vi "FilterByMatchingString.vi"(6 "AND Condition?":bool, 8 "error in (no error)":errorcluster, 9 "Target filter":refnum<class "CItemMatch.lvclass">, 10 "Source filter":refnum<class "CItemMatch.lvclass">, 11 "CDependencyList in":refnum<class "CDependencyList.lvclass">) -> (0 "error out":errorcluster, 3 "CDependencyList out":refnum<class "CDependencyList.lvclass">)   [LabVIEW 2020, in "DependencyInspection.lvlib" / "CDependencyList.lvclass"]
uses:
  CDependencyList.lvclass
  LabVIEWObjectInterfaces/ILabVIEWItem/ILabVIEWItem.lvclass
  LabVIEWObjectFactory/LabVIEWObjectFactory.lvlib
  CItemMatch/CItemMatch.lvclass
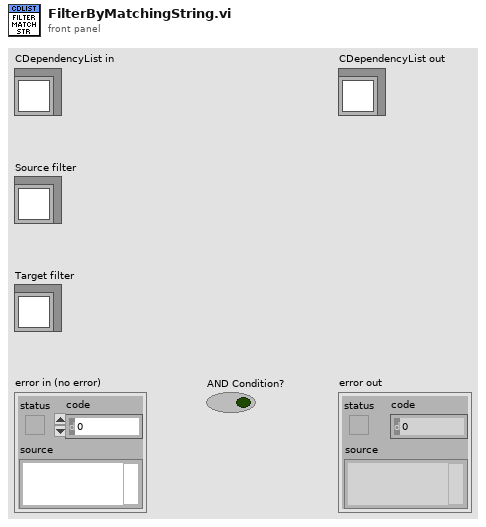
[diagram p1: front panel]
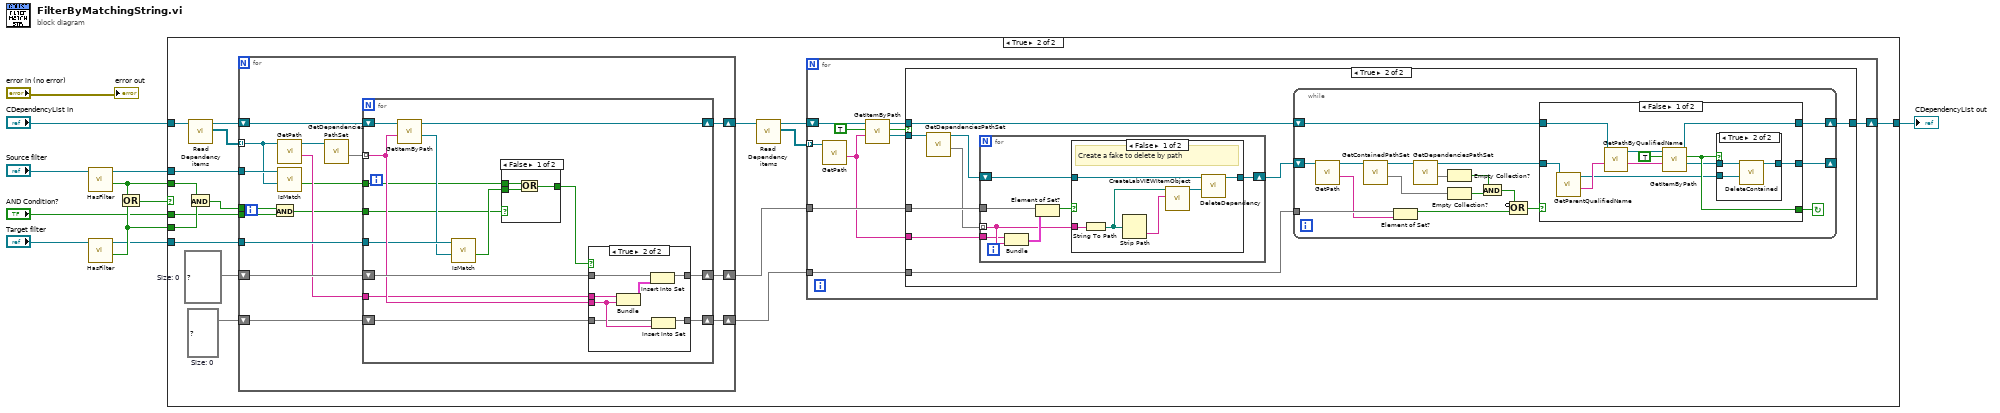
[diagram p0: block diagram]
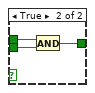
[diagram p3: hidden frame]
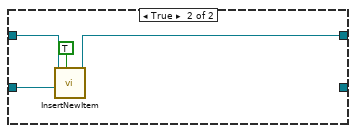
[diagram p8: hidden frame]
diagram:
  n1 = call-dynamic "HasFilter.vi"("CItemMatch in"="Source filter") -> ("Has filter?"=w7:bool, "CItemMatch out"=w5:refnum<class "CItemMatch.lvclass">)  [unwired: 8 in, 1 out]
  n2 = call-dynamic "HasFilter.vi"("CItemMatch in"="Target filter") -> ("Has filter?"=w4:bool, "CItemMatch out"=w2:refnum<class "CItemMatch.lvclass">)  [unwired: 8 in, 1 out]
  n3 = Or(x=w7, y=w4) -> (x .or. y?=w8:bool)
  n4 = case shown="True" w8 {
    tunnel: "CDependencyList in" -> [w12 w29]
    tunnel: w2 -> [_ w25]
    tunnel: w5 -> [_ w24]
    tunnel: [w12 w19] -> w9
    tunnel: w7 -> [_ w18]
    tunnel: w4 -> [_ w17]
    tunnel: "AND Condition?" -> [_ w13]
    frame False {
    }
    frame True {
      w16 = set{string} {}  # Size: 0
      w23 = set{cluster{"Source":string, "Target":string}} {}  # Size: 0
      n5 = call-dynamic "Read Dependency items.vi"("CDependencyList in"=w29) -> ("Dependency items"=w28:refnum<class "ILabVIEWItem.lvclass">[], "CDependencyList out"=w27:refnum<class "CDependencyList.lvclass">)  [unwired: 9 in]
      n6 = And(x=w18, y=w17) -> (x .and. y?=w14:bool)
      n7 = for {
        tunnel: w28 -> [w37] mode=indexing
        shift-right: [w43] -> w26
        shift-left: w27 -> [w45]
        tunnel: w25 -> [w44]
        tunnel: w24 -> [w38]
        shift-right: [w42] -> w20
        shift-left: w23 -> [w41]
        shift-right: [w40] -> w15
        shift-left: w16 -> [w39]
        tunnel: w14 -> [w30]
        tunnel: w13 -> [w32]
        n8 = And(x=w30, y=w32) -> (x .and. y?=w31:bool)
        n9 = call-dynamic "GetPath.vi"("ILabVIEWItem in"=w37) -> ("Path"=w34:string, "ILabVIEWItem out"=w35:refnum<class "ILabVIEWItem.lvclass">)  [unwired: 8 in, 1 out]
        n10 = call-dynamic "IsMatch.vi"("Item to match"=w37, "CItemMatch in"=w38) -> ("Is match?"=w33:bool)  [unwired: 7 in, 2 out]
        n11 = call-dynamic "GetDependenciesPathSet.vi"("ILabVIEWItem in"=w35) -> ("Dependencies"=w36:set{string})  [unwired: 8 in, 2 out]
        n12 = for {
          tunnel: w36 -> [w55] mode=indexing
          shift-right: [w58] -> w43
          shift-left: w45 -> [w59]
          tunnel: w44 -> [w51]
          shift-right: [w56] -> w42
          shift-left: w41 -> [w57]
          tunnel: w34 -> [w54]
          shift-right: [w53] -> w40
          shift-left: w39 -> [w52]
          tunnel: w33 -> [w48]
          tunnel: w31 -> [w47]
          n13 = call-dynamic "GetItemByPath.vi"("Path"=w55, "CDependencyList in"=w59) -> ("ILabVIEWItem"=w50:refnum<class "ILabVIEWItem.lvclass">, "CDependencyList out"=w58:refnum<class "CDependencyList.lvclass">)  [unwired: 6 in, 2 out]
          n14 = call-dynamic "IsMatch.vi"("Item to match"=w50, "CItemMatch in"=w51) -> ("Is match?"=w49:bool)  [unwired: 7 in, 2 out]
          n15 = case shown="False" w47 {
            tunnel: w49 -> [w62 w64]
            tunnel: w48 -> [w61 w65]
            tunnel: [w60 w63] -> w46
            frame False {
              n16 = Or(x=w61, y=w62) -> (x .or. y?=w60:bool)
            }
            frame True {
              n17 = And(x=w65, y=w64) -> (x .and. y?=w63:bool)
            }
          }
          n18 = case shown="True" w46 {
            tunnel: w57 -> [w67 w73]
            tunnel: [w67 w74] -> w56
            tunnel: w55 -> [_ w70]
            tunnel: w54 -> [_ w72]
            tunnel: [w66 w69] -> w53
            tunnel: w52 -> [w66 w68]
            frame False {
            }
            frame True {
              n19 = Bundle("Path"=w72, "Path"=w70) -> (w71:cluster{"Path":string, "Path":string})  [unwired: 1 in]
              n20 = Insert Into Set(10:w71, 11:w73) -> (3:w74:set{cluster{"Source":string, "Target":string}})  [unwired: 1 out]
              n21 = Insert Into Set(10:w70, 11:w68) -> (3:w69:set{string})  [unwired: 1 out]
            }
          }
        }
      }
      n22 = call-dynamic "Read Dependency items.vi"("CDependencyList in"=w26) -> ("Dependency items"=w21:refnum<class "ILabVIEWItem.lvclass">[], "CDependencyList out"=w22:refnum<class "CDependencyList.lvclass">)  [unwired: 9 in]
      n23 = for {
        shift-right: [w79] -> w19
        shift-left: w22 -> [w83]
        tunnel: w21 -> [w82] mode=indexing
        tunnel: w20 -> [w78]
        tunnel: w15 -> [w75]
        n24 = call-dynamic "GetPath.vi"("ILabVIEWItem in"=w82) -> ("Path"=w76:string)  [unwired: 8 in, 2 out]
        n25 = call-dynamic "GetItemByPath.vi"("Path"=w76, "Remove?"=TRUE, "CDependencyList in"=w83) -> ("ILabVIEWItem"=w80:refnum<class "ILabVIEWItem.lvclass">, "key found?"=w77:bool, "CDependencyList out"=w81:refnum<class "CDependencyList.lvclass">)  [unwired: 5 in, 1 out]
        n26 = case shown="True" w77 {
          tunnel: w81 -> [w85 w90]
          tunnel: w80 -> [_ w93]
          tunnel: [w85 w94] -> w79
          tunnel: w78 -> [_ w91]
          tunnel: w76 -> [_ w87]
          tunnel: w75 -> [_ w86]
          frame False {
          }
          frame True {
            n27 = call-dynamic "GetDependenciesPathSet.vi"("ILabVIEWItem in"=w93) -> ("Dependencies"=w89:set{string}, "ILabVIEWItem out"=w88:refnum<class "ILabVIEWItem.lvclass">)  [unwired: 8 in, 1 out]
            n28 = for {
              tunnel: w89 -> [w96] mode=indexing
              tunnel: w91 -> [w101]
              shift-right: [w98] -> w92
              shift-left: w88 -> [w99]
              tunnel: w87 -> [w95]
              n29 = Bundle("Path"=w95, "Path"=w96) -> (w97:cluster{"Path":string, "Path":string})  [unwired: 1 in]
              n30 = Element of Set?(10:w97, 11:w101) -> (3:w100:bool)
              n31 = case shown="False" w100 {
                tunnel: w99 -> [w107 w108]
                tunnel: [w106 w108] -> w98
                tunnel: w96 -> [w104 _]
                frame False {
                  # "Create a fake to delete by path"
                  n32 = String To Path(string=w104) -> (path=w102:path)
                  n33 = Strip Path(path=w102) -> (name=w103:string)  [unwired: 1 out]
                  n34 = call "CreateLabVIEWItemObject.vi"("delimited name"=w103, "SubVI path"=w102) -> ("ILabVIEWItem"=w105:refnum<class "ILabVIEWItem.lvclass">)  [unwired: 8 in, 1 out]
                  n35 = call-dynamic "DeleteDependency.vi"("Item to depend on"=w105, "ILabVIEWItem in"=w107) -> ("ILabVIEWItem out"=w106:refnum<class "ILabVIEWItem.lvclass">)  [unwired: 8 in, 1 out]
                }
                frame True {
                }
              }
            }
            n36 = while {
              shift-right: [w120] -> w94
              shift-left: w90 -> [w123]
              shift-right: [w119] -> _
              shift-left: w92 -> [w117]
              tunnel: w86 -> [w115]
              stop <- w118 continue-if-true
              n37 = call-dynamic "GetPath.vi"("ILabVIEWItem in"=w117) -> ("Path"=w110:string, "ILabVIEWItem out"=w116:refnum<class "ILabVIEWItem.lvclass">)  [unwired: 8 in, 1 out]
              n38 = call-dynamic "GetContainedPathSet.vi"("ILabVIEWItem in"=w116) -> ("Contained"=w121:set{string}, "ILabVIEWItem out"=w122:refnum<class "ILabVIEWItem.lvclass">)  [unwired: 8 in, 1 out]
              n39 = Element of Set?(10:w110, 11:w115) -> (3:w112:bool)
              n40 = call-dynamic "GetDependenciesPathSet.vi"("ILabVIEWItem in"=w122) -> ("Dependencies"=w125:set{string}, "ILabVIEWItem out"=w124:refnum<class "ILabVIEWItem.lvclass">)  [unwired: 8 in, 1 out]
              n41 = Empty Collection?(1:w125) -> (0:w113:bool)
              n42 = Empty Collection?(1:w121) -> (0:w114:bool)
              n43 = And(x=w113, y=w114) -> (x .and. y?=w111:bool)
              n44 = Compound Arithmetic op=OR(invert w111, w112) -> (w109:bool)
              n45 = case shown="False" w109 {
                tunnel: w124 -> [w128 w142]
                tunnel: w123 -> [w127 w143]
                tunnel: [w126 w141] -> w120
                tunnel: [w132 _] -> w118
                tunnel: [w129 _] -> w119
                frame False {
                  n46 = call-dynamic "GetParentQualifiedName.vi"("ILabVIEWItem in"=w128) -> ("Name"=w136:string, "ILabVIEWItem out"=w131:refnum<class "ILabVIEWItem.lvclass">)  [unwired: 8 in, 1 out]
                  n47 = call-dynamic "GetPathByQualifiedName.vi"("Qualified name"=w136, "CDependencyList in"=w127) -> ("Path"=w133:string, "CDependencyList out"=w134:refnum<class "CDependencyList.lvclass">)  [unwired: 6 in, 2 out]
                  n48 = call-dynamic "GetItemByPath.vi"("Path"=w133, "Remove?"=TRUE, "CDependencyList in"=w134) -> ("ILabVIEWItem"=w130:refnum<class "ILabVIEWItem.lvclass">, "key found?"=w132:bool, "CDependencyList out"=w126:refnum<class "CDependencyList.lvclass">)  [unwired: 5 in, 1 out]
                  n49 = case shown="True" w132 {
                    tunnel: w130 -> [w137 w140]
                    tunnel: w131 -> [_ w139]
                    tunnel: [w137 w138] -> w129
                    frame False {
                    }
                    frame True {
                      n50 = call-dynamic "DeleteContained.vi"("Item to contain"=w139, "ILabVIEWItem in"=w140) -> ("ILabVIEWItem out"=w138:refnum<class "ILabVIEWItem.lvclass">)  [unwired: 8 in, 1 out]
                    }
                  }
                }
                frame True {
                  n51 = call-dynamic "InsertNewItem.vi"("Replace?"=TRUE, "ILabVIEWItem in"=w142, "CDependencyList in"=w143) -> ("CDependencyList out"=w141:refnum<class "CDependencyList.lvclass">)  [unwired: 6 in, 2 out]
                }
              }
            }
          }
        }
      }
    }
  }
  "CDependencyList out" <- w9
  "error out" <- "error in (no error)"
